vi "TPNT_GetByType.vi"(10 "type":string="ALL") -> (2 "full out":string)   [LabVIEW 2016]
uses:
  TPNT_CoreFunction.ctl
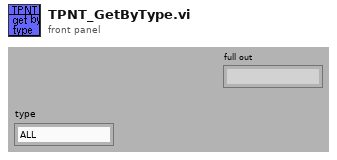
[diagram p1: front panel]
types:
  T1 = typedef "TPNT_CoreFunction.ctl" = enum16{"Reset", "Register", "Get Data", "Set Data", "Unregister", "Test", "Get Objects"}
  T2 = typedef "TPNT_Refnum.ctl" = refnum<vi>
  T3 = typedef "TPNT_TP.ctl" = cluster{"name":string, "type":string, "algor":string[], "update_rate":sgl, "Limits":T4, "Samples":T5, "next_update":u32, "Status":string, "monitor":bool, "error":bool, "Log":T6, "permissions":string, "ID":string}
  T4 = typedef "TPNT_Limits.ctl" = cluster{"Alarm Type":string, "Lower ":dbl, "Upper":dbl, "Nominal":dbl, "outrange":bool, "Check":bool, "latch":bool, "level":string}
  T5 = typedef "TPNT_Samples.ctl" = cluster{"samples":i32, "counter":i32, "Values":dbl[], "Current Value":string, "filter":string, "precision":u8}
  T6 = typedef "TPNT_Log.ctl" = cluster{"log":bool, "file":path, "type":string, "format":string, "updaterate":dbl, "nex_update":u32, "mode":string}
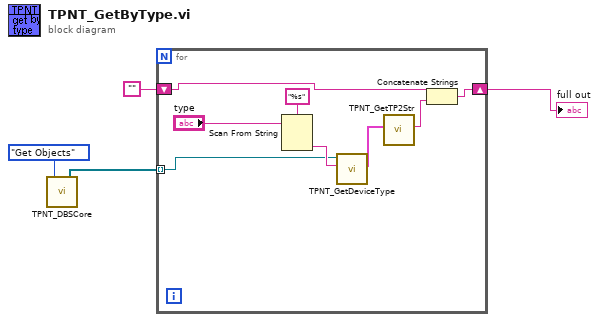
[diagram p0: block diagram]
diagram:
  n1 = call "TPNT_DBSCore.vi"("Function (Get Data)"=TPNT_CoreFunction."Get Objects") -> ("Objects"=w3:T2[])  [unwired: 4 in, 14 out]
  n2 = for {
    tunnel: w3 -> [w9] mode=indexing
    shift-right: [w6] -> w1
    shift-left: "" -> [w5]
    n3 = Scan From String(format string="%s", input string="type") -> (output 1=w11:string)  [unwired: 2 in, 4 out]
    n4 = call "TPNT_GetDeviceType.vi"("tptype"=w11, "Object Refnum In"=w9) -> ("Type"=w12:T3[])  [unwired: 1 in, 8 out]
    n5 = call "TPNT_GetTP2Str.vi"("TPs"=w12) -> ("String"=w7:string)  [unwired: 1 in, 9 out]
    n6 = Concatenate Strings(w5, w7) -> (w6:string)
  }
  "full out" <- w1
